vi "Set Thermostat Target Temperature.vi"   [LabVIEW 2013, in "LVH-Nest.lvlib"]
uses:
  LVH-Nest.lvlib
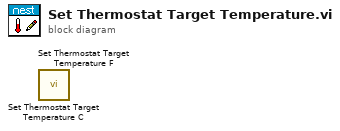
[diagram p0: block diagram]
diagram:
  n1 = call "Set Thermostat Target Temperature C.vi"() -> ()  [unwired: 10 in, 2 out]
  n2 = call "Set Thermostat Target Temperature F.vi"() -> ()  [unwired: 10 in, 2 out]
